vi "Timer(SubVI).vi"(9 "Reset after time reached?":bool, 10 "Time to count up to":dbl format="%#_13g", 11 "Reset?":bool) -> (2 "Time reached?":bool, 3 "Current time":dbl)   [LabVIEW 2015]
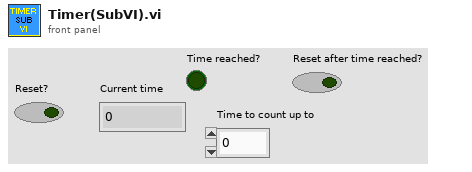
[diagram p1: front panel]
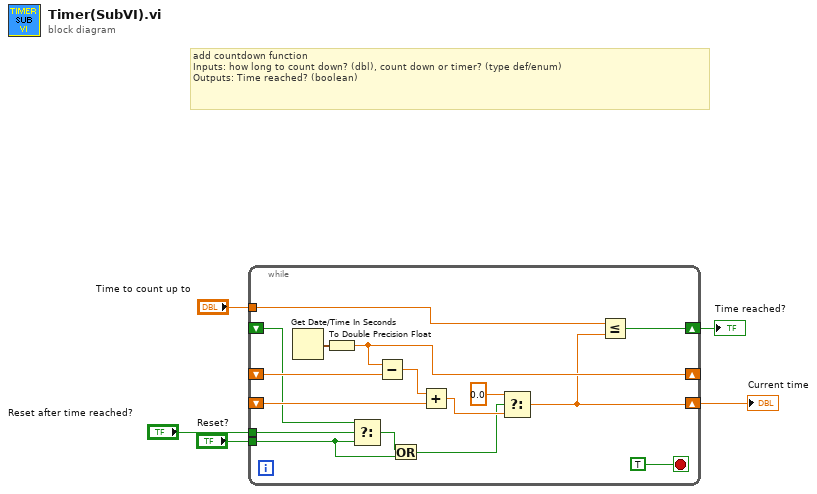
[diagram p0: block diagram]
diagram:
  # "add countdown function\nInputs: how long to count down? (dbl), count down or timer? (type def/enum)\nOutputs: Time reached? (boolean)"
  n1 = while {
    shift-right: [w20] -> _
    shift-left: _ -> [w19]
    shift-right: [w12] -> w4
    shift-left: _ -> [w17]
    tunnel: "Reset?" -> [w8]
    tunnel: "Reset after time reached?" -> [w10]
    tunnel: "Time to count up to" -> [w13]
    shift-right: [w11] -> w2
    shift-left: _ -> [w9]
    stop <- TRUE stop-if-true
    n2 = Get Date/Time In Seconds() -> (seconds since 1Jan1904=w21:timestamp)
    n3 = To Double Precision Float(number=w21) -> (double precision float=w20:dbl)
    n4 = Select(t=w9, s=w10, f=w8) -> (s? t:f=w7:bool)
    n5 = Subtract(x=w20, y=w19) -> (x-y=w18:dbl)
    n6 = Or(x=w7, y=w8) -> (x .or. y?=w6:bool)
    n7 = Add(x=w18, y=w17) -> (x+y=w15:dbl)
    n8 = Select(t=0.0, s=w6, f=w15) -> (s? t:f=w12:dbl)
    n9 = Less Or Equal?(x=w13, y=w12) -> (x <= y?=w11:bool)
  }
  "Current time" <- w4
  "Time reached?" <- w2
